vi "Common Issues.vi"(8 "error in (no error)":errorcluster, 11 "ColumnPanel in":refnum<class "ColumnPanel.lvclass">) -> (0 "error out":errorcluster, 2 "Issues":string[](array[string]), 3 "ColumnPanel out":refnum<class "ColumnPanel.lvclass">)   [LabVIEW 2020, in "Conditum-Tools.lvlib" / "ColumnPanel.lvclass"]
uses:
  ColumnPanel.lvclass
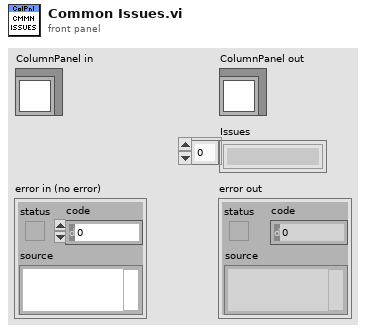
[diagram p1: front panel]
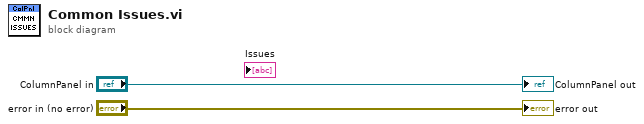
[diagram p0: block diagram]
diagram:
  "error out" <- "error in (no error)"
  "ColumnPanel out" <- "ColumnPanel in"
